vi "bigEncoder.vi"(4 "Positive Direction":bool, 5 "ForceReset":bool, 6 "Reset C State":bool, 7 "C":bool, 8 "Reset B State":bool, 9 "Reset A State":bool, 10 "B":bool, 11 "A":bool) -> (1 "JumpBy2Error":i16, 2 "Position":i32)   [LabVIEW 2010, in "KevLib01.lvlib"]
uses:
  KevLib01.lvlib
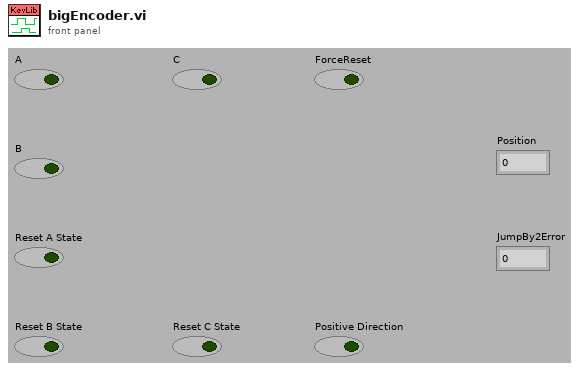
[diagram p1: front panel]
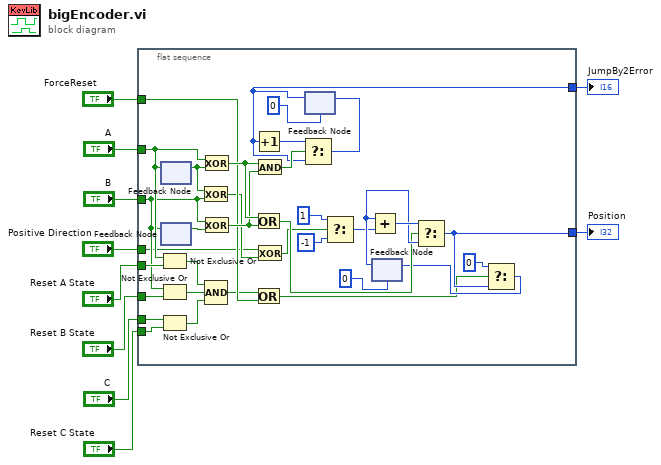
[diagram p0: block diagram]
diagram:
  n1 = flat-sequence {
    tunnel: "A" -> [w23]
    tunnel: "B" -> [w21]
    tunnel: [w28] -> w8
    tunnel: [w31] -> w7
    tunnel: "ForceReset" -> [w25]
    tunnel: "Reset A State" -> [w24]
    tunnel: "Reset B State" -> [w22]
    tunnel: "Reset C State" -> [w20]
    tunnel: "C" -> [w19]
    tunnel: "Positive Direction" -> [w11]
    frame #0 {
      n2 = Not Exclusive Or(1:w24, 2:w23) -> (0:w18:bool)
      n3 = Not Exclusive Or(1:w22, 2:w21) -> (0:w17:bool)
      n4 = Not Exclusive Or(1:w20, 2:w19) -> (0:w16:bool)
      n5 = feedback-in #1(w23) -> ()
      n6 = feedback #1() -> (w43:bool)  [unwired: 1 out]
      n7 = feedback-in #2(w21) -> ()
      n8 = feedback #2() -> (w44:bool)  [unwired: 1 out]
      n9 = Exclusive Or(1:w21, 2:w43) -> (0:w13:bool)
      n10 = Exclusive Or(1:w43, 2:w23) -> (0:w37:bool)
      n11 = Exclusive Or(1:w44, 2:w21) -> (0:w36:bool)
      n12 = Compound Arithmetic op=AND(w18, w17, w16) -> (w15:bool)
      n13 = Or(x=w37, y=w36) -> (x .or. y?=w30:bool)
      n14 = Or(x=w15, y=w25) -> (x .or. y?=w14:bool)
      n15 = And(x=w37, y=w36) -> (x .and. y?=w34:bool)
      n16 = Exclusive Or(1:w13, 2:w11) -> (0:w12:bool)
      n17 = feedback #3(i16 0) -> (w31:i16)
      n18 = Increment(x=w31) -> (x+1=w33:i16)
      n19 = Select(t=w33, s=w34, f=w31) -> (s? t:f=w32:i16)
      n20 = feedback-in #3(w32) -> ()
      n21 = Select(t=1, s=w12, f=-1) -> (s? t:f=w29:i32)
      n22 = feedback #4(0) -> (w38:i32)
      n23 = Add(x=w38, y=w29) -> (x+y=w42:i32)
      n24 = Select(t=w42, s=w30, f=w38) -> (s? t:f=w28:i32)
      n25 = Select(t=0, s=w14, f=w28) -> (s? t:f=w26:i32)
      n26 = feedback-in #4(w26) -> ()
    }
  }
  "Position" <- w8
  "JumpBy2Error" <- w7
